vi "VelocityFix.vi"(9 "Tolerance":dbl=1e-05, 10 "Smooth Vel":dbl[][](array[numeric]), 11 "Orig Vel":dbl[][](array[numeric])) -> (3 "Fixed Vel":dbl[][](array[numeric]))   [LabVIEW 2016]
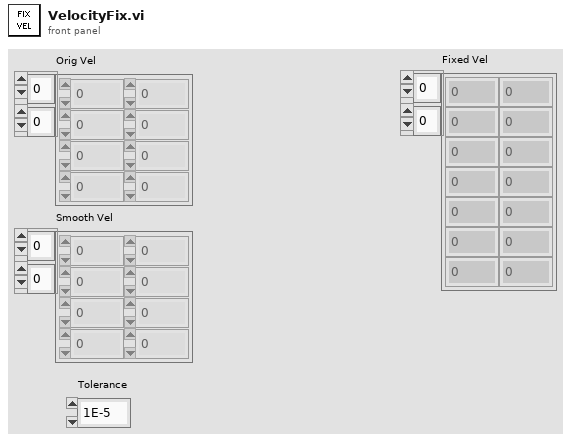
[diagram p1: front panel]
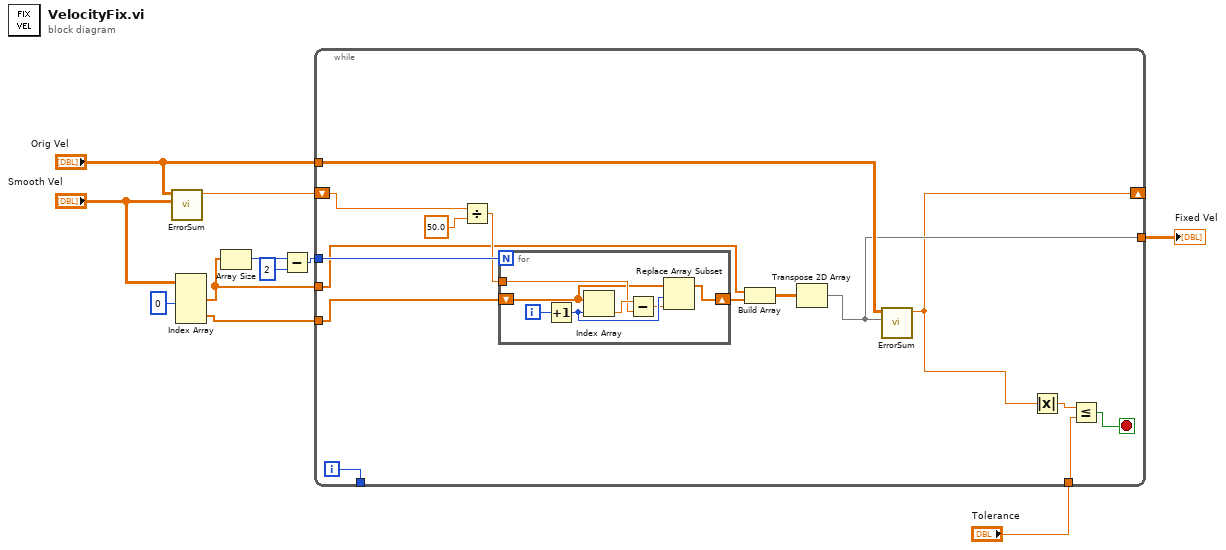
[diagram p0: block diagram]
diagram:
  n1 = call "ErrorSum.vi"("Smooth Vel"="Smooth Vel", "Orig Vel"="Orig Vel") -> ("Difference"=w10:dbl)  [unwired: 9 in]
  n2 = Index Array(array="Smooth Vel", index (col) #1=0 ("disabled index (col)")) -> (element #1=w6:dbl[], element #2=w7:dbl[])  [unwired: 3 in]
  n3 = Array Size(array=w6) -> (size(s)=w3:i32)
  n4 = Subtract(x=w3, y=2) -> (x-y=w1:i32)
  n5 = while {
    tunnel: "Tolerance" -> [w25]
    tunnel: w1 -> [w22]
    tunnel: w7 -> [w19]
    tunnel: w6 -> [w18]
    tunnel: "Orig Vel" -> [w17]
    tunnel: [w15] -> w4
    shift-right: [w13] -> _
    shift-left: w10 -> [w14]
    tunnel: [w12] -> _
    i -> [w12]
    stop <- w26 stop-if-true
    n6 = Divide(x=w14, y=50.0) -> (x/y=w21:dbl)
    n7 = for {
      N: w22 -> [_]
      tunnel: w21 -> [w31]
      shift-right: [w27] -> w20
      shift-left: w19 -> [w30]
      i -> [w33]
      n8 = Increment(x=w33) -> (x+1=w29:i32)
      n9 = Index Array(array=w30, index=w29) -> (element=w32:dbl)
      n10 = Subtract(x=w32, y=w31) -> (x-y=w28:dbl)
      n11 = Replace Array Subset(array=w30, new element=w28, index=w29) -> (w27:dbl[])
    }
    n12 = Build Array(w18, w20) -> (w16:dbl[][])
    n13 = Transpose 2D Array(2D array=w16) -> (transposed array=w15:dbl[][])
    n14 = call "ErrorSum.vi"("Smooth Vel"=w15, "Orig Vel"=w17) -> ("Difference"=w13:dbl)  [unwired: 9 in]
    n15 = Absolute Value(x=w13) -> (abs(x)=w24:dbl)
    n16 = Less Or Equal?(x=w24, y=w25) -> (x <= y?=w26:bool)
  }
  "Fixed Vel" <- w4
